vi "led_strobe.vi"(0 "Device Handle":u32, 5 "Channel":i32, 7 "Wait Time":u32, 9 "REPEATS":u32, 11 "Current":u32, 12 "Pulse Length":u32) -> (4 "Device Handle Out":u32, 6 "Channel Out":i32)   [LabVIEW 2013]
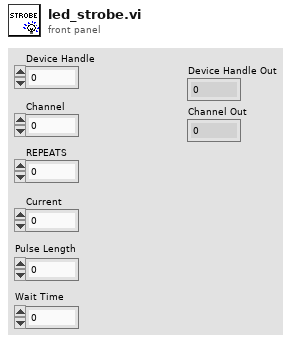
[diagram p1: front panel]
types:
  T1 = enum16{"Set Mode", "Set  Current Max", "Set Current "}
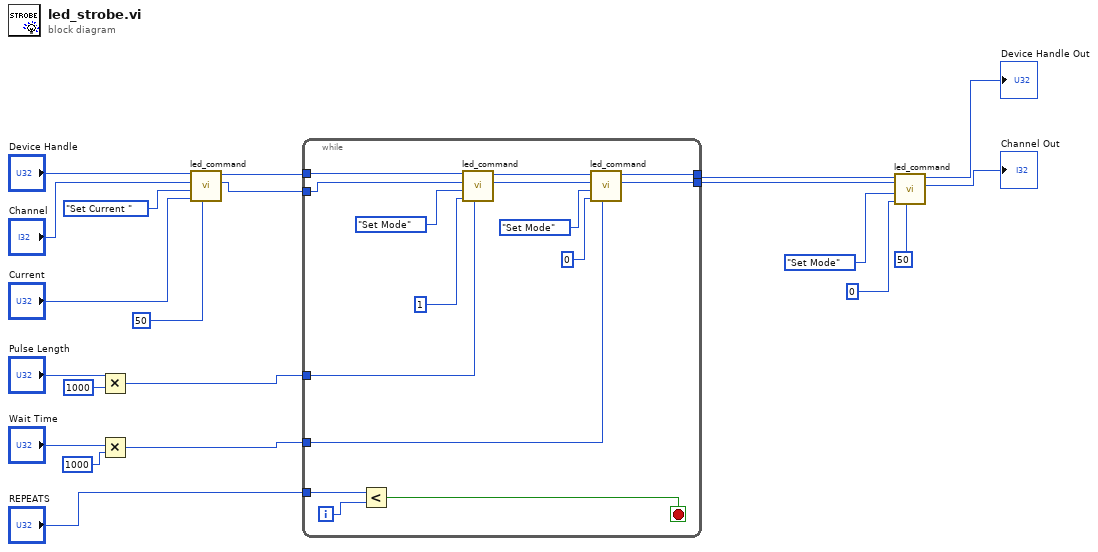
[diagram p0: block diagram]
diagram:
  n1 = Multiply(x="Pulse Length", y=u32 1000) -> (x*y=w19:u32)
  n2 = Multiply(x="Wait Time", y=u32 1000) -> (x*y=w9:u32)
  n3 = call "led_command.vi"("milliseconds to wait"=u32 50, "INPUT"="Current", "COMMANDS"=T1."Set Current ", "Channel"="Channel", "Device Handle"="Device Handle") -> ("Channel Out"=w4:i32, "Device Handle Out"=w7:u32)  [unwired: 5 in]
  n4 = while {
    tunnel: "REPEATS" -> [w36]
    tunnel: w19 -> [w33]
    tunnel: [w28] -> w17
    tunnel: [w27] -> w1
    tunnel: w7 -> [w24]
    tunnel: w9 -> [w26]
    tunnel: w4 -> [w23]
    i -> [w35]
    stop <- w22 stop-if-true
    n5 = Less?(x=w36, y=w35) -> (x < y?=w22:bool)
    n6 = call "led_command.vi"("milliseconds to wait"=w33, "INPUT"=u32 1, "COMMANDS"=T1."Set Mode", "Channel"=w23, "Device Handle"=w24) -> ("Channel Out"=w31:i32, "Device Handle Out"=w32:u32)  [unwired: 5 in]
    n7 = call "led_command.vi"("milliseconds to wait"=w26, "INPUT"=u32 0, "COMMANDS"=T1."Set Mode", "Channel"=w31, "Device Handle"=w32) -> ("Channel Out"=w27:i32, "Device Handle Out"=w28:u32)  [unwired: 5 in]
  }
  n8 = call "led_command.vi"("milliseconds to wait"=u32 50, "INPUT"=u32 0, "COMMANDS"=T1."Set Mode", "Channel"=w1, "Device Handle"=w17) -> ("Channel Out"=→"Channel Out":i32, "Device Handle Out"=→"Device Handle Out":u32)  [unwired: 5 in]
